vi "Play Sound.vi"(8 "error in (no error)":errorcluster, 10 "File Name":string="jeopardy-board-sms.wav", 11 "Controller in":refnum<class "Controller.lvclass">) -> (0 "error out":errorcluster, 3 "Controller out":refnum<class "Controller.lvclass">)   [LabVIEW 2021, in "Controller.lvlib" / "Controller.lvclass"]
uses:
  Controller.lvclass
  C:/Program Files/National Instruments/LabVIEW 2024/vi.lib/ActorFramework/Actor/Actor.lvclass
  Controller.lvclass/Controller.ctl
  Sounds/Sounds/Sounds.lvclass
  Sounds/Sounds/Sounds.lvclass/Sounds.ctl
  <vilib>/ActorFramework/Actor/Actor.lvclass
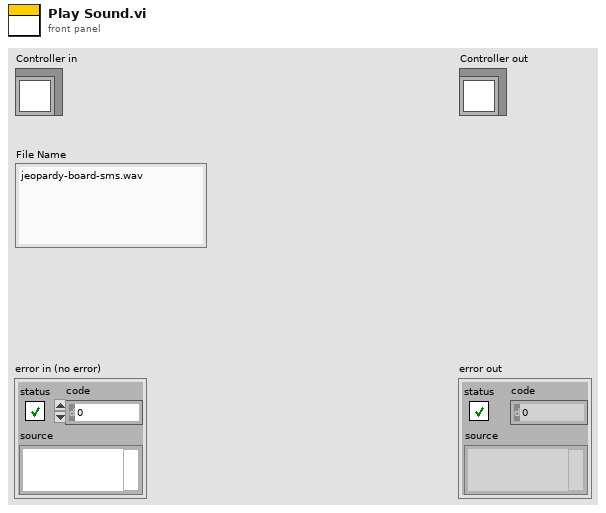
[diagram p1: front panel]
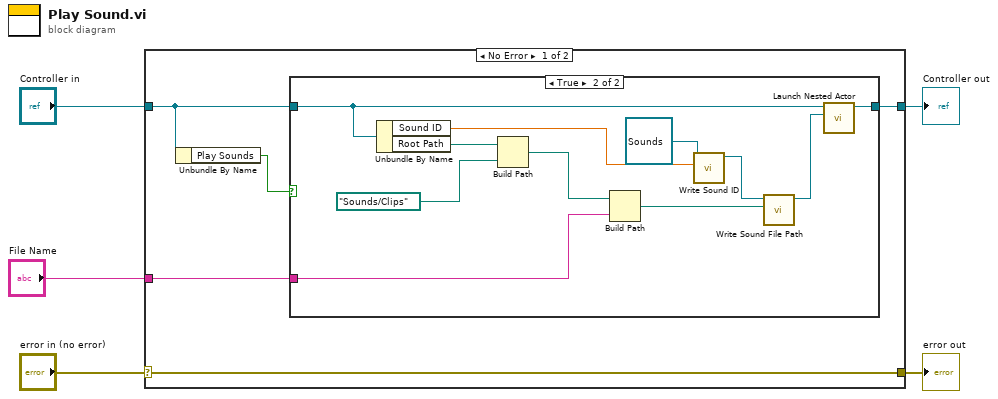
[diagram p0: block diagram]
diagram:
  n1 = case shown="No Error" "error in (no error)" {
    selector: "error in (no error)" -> [w10 w24]
    tunnel: [w10 w24] -> w4
    tunnel: [w9 w23] -> w2
    tunnel: "Controller in" -> [w7 w23]
    tunnel: "File Name" -> [w8 _]
    frame No Error {
      n2 = Unbundle By Name(w7) -> ("Play Sounds"=w6:bool)
      n3 = case shown="True" w6 {
        tunnel: [w11 w22] -> w9
        tunnel: w8 -> [_ w16]
        tunnel: w7 -> [w11 w15]
        frame False {
        }
        frame True {
          n4 = Unbundle By Name(w15) -> ("Sound ID"=w12:dbl, "Root Path"=w20:path)
          n5 = Build Path(base path=w20, name or relative path=path "Sounds/Clips") -> (appended path=w18:path)
          n6 = Build Path(base path=w18, name or relative path=w16) -> (appended path=w17:path)
          n7 = call "Write Sound ID.vi"("Sound ID"=w12, "Sounds in"=refnum<class "Sounds.lvclass"> refnum ("Sounds.lvlib:Sounds.lvclass")) -> ("Sounds out"=w13:refnum<class "Sounds.lvclass">)  [unwired: 8 in, 1 out]
          n8 = call "Write Sound File Path.vi"("Sound File Path"=w17, "Sounds in"=w13) -> ("Sounds out"=w21:refnum<class "Sounds.lvclass">)  [unwired: 8 in, 1 out]
          n9 = call <vilib>:"Launch Nested Actor.vi"("Nested Actor"=w21, "Caller Actor in"=w15) -> ("Caller Actor out"=w22:refnum<class "Controller.lvclass">)  [unwired: 7 in, 2 out]
        }
      }
    }
    frame Error {
    }
  }
  "error out" <- w4
  "Controller out" <- w2
